vi "Read Config.vi"(8 "error in (no error)":errorcluster, 10 "Resource In":variant, 11 "Analyze Parameter Energy per Count in":refnum<class "Analyze Parameter Energy per Count.lvclass">) -> (0 "error out":errorcluster, 2 "Resource Out":variant, 3 "Analyze Parameter Energy per Count out":refnum<class "Analyze Parameter Energy per Count.lvclass">)   [LabVIEW 2020, in "Analyze Parameter Energy per Count.lvclass"]
uses:
  Analyze Parameter Energy per Count.lvclass
  C:/POLARIS Programme/POLARIS-AS-3-Cams/Submodules/HIJ Vision/Analyze/Analyze Parameter/Analyze Parameter Base/Analyze Parameter Base.lvclass
  <vilib>/Utility/config.llb/Config Data RefNum.ctl
  Analyze Parameter Energy per Count.lvclass/Analyze Parameter Energy per Count.ctl
  <vilib>/Utility/config.llb/Read Key (Double).vi
  <vilib>/Utility/config.llb/NI_LVConfig.lvlib
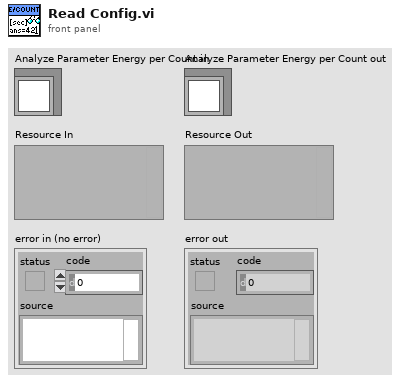
[diagram p1: front panel]
types:
  T1 = typedef "NI_LVConfig.lvlib/Config Data RefNum.ctl" = refnum<k1>
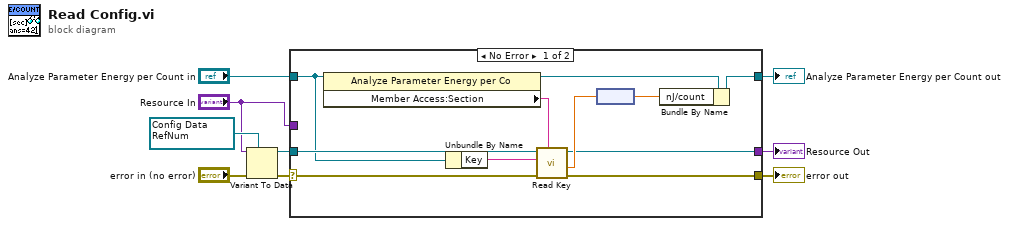
[diagram p0: block diagram]
diagram:
  w6 = T1 refnum items=["config data"] ("refnum")
  n1 = Variant To Data(error in="error in (no error)", type=w6, Variant="Resource In") -> (data=w8:T1, error out=w9:errorcluster)
  n2 = case shown="No Error" w9 {
    selector: w9 -> [w14 w22]
    tunnel: w8 -> [w20 _]
    tunnel: "Analyze Parameter Energy per Count in" -> [w15 w21]
    tunnel: [w18 w21] -> w3
    tunnel: [w12 w23] -> w2
    tunnel: [w11 w22] -> w1
    tunnel: "Resource In" -> [_ w23]
    frame No Error {
      n3 = property class="Analyze Parameter Energy per Co"(reference=w15) -> (reference out=w16:refnum<class "Analyze Parameter Energy per Count.lvclass">, "Member Access:Section"=w13:string)  [unwired: 1 in, 1 out]
      n4 = Unbundle By Name(w15) -> ("Key"=w17:string)
      n5 = call-poly <vilib>:"Read Key.vi"("section"=w13, "error in (no error)"=w14, "key"=w17, "refnum"=w20) -> ("error out"=w11:errorcluster, "value"=w19:dbl, "refnum out"=w12:T1)  [unwired: 4 in, 1 out]
      n6 = node(w19) -> (w10:dbl[unit])
      n7 = Bundle By Name(cluster=w16, "nJ/count"=w10) -> (w18:refnum<class "Analyze Parameter Energy per Count.lvclass">)
    }
    frame Error {
    }
  }
  "error out" <- w1
  "Analyze Parameter Energy per Count out" <- w3
  "Resource Out" <- w2
